vi "Configure Clock Recovery Method.vi"(0 "VISA resource name":refnum<visa-resource-name>, 1 "Clock":T1 {"Clock Edge (0: Rising)" items=["Rising", "Falling", "Both"]}, 2 "Track Frequency (2.5E+9 Hz)":dbl, 5 "Measurement Source (1: Channel 1)":i32(ring) items=["Channel 1", "Channel 2", "Channel 3", "Channel 4", "Function 1", "Function 2", "Function 3", "Function 4", "Memory 1", "Memory 2", "Memory 3", "Memory 4"], 7 "Clock Recovery Method (4: Constant Frequency)":i32(ring) items=["PCI Express", "Fibre Channel", "First Order PLL", "Second Order PLL", "Constant Frequency", "Explicit Clock", "Explicit First Order PLL", "Explicit Second Order PLL"], 9 "Data Rate and Bandwidth":T2 {"Data Bits (0: Both)" items=["Both", "Deemphasis", "Transition"]; "Data Rate Type (0: Fully Automatic)" items=["Fully Automatic", "Semi-Automatic", "Manual"]}, 11 "error in (no error)":errorcluster, 12 "Fibre Channel (0: FC1063)":i32(ring) items=["FC1063", "FC2125", "FC425"], 13 "Damping Factor (1 bits/s)":dbl format="%#.3g") -> (4 "VISA resource name out":refnum<visa-resource-name>, 15 "error out":errorcluster)   [LabVIEW 2009, in "Agilent 8000 Series.lvlib"]
doc: "Configures the clock recovery method parameters."
uses:
  Agilent 8000 Series.lvlib
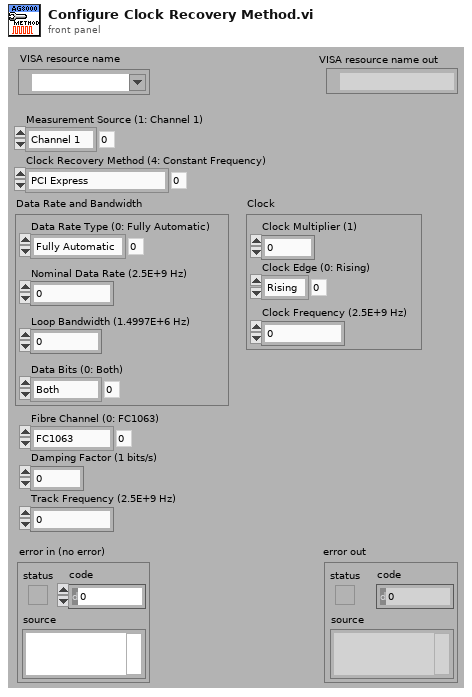
[diagram p1: front panel]
types:
  T1 = cluster{"Clock Edge (0: Rising)":i32, "Clock Multiplier (1)":i32, "Clock Frequency (2.5E+9 Hz)":dbl}
  T2 = cluster{"Nominal Data Rate (2.5E+9 Hz)":dbl, "Loop Bandwidth (1.4997E+6 Hz)":dbl, "Data Rate Type (0: Fully Automatic)":i32, "Data Bits (0: Both)":i32}
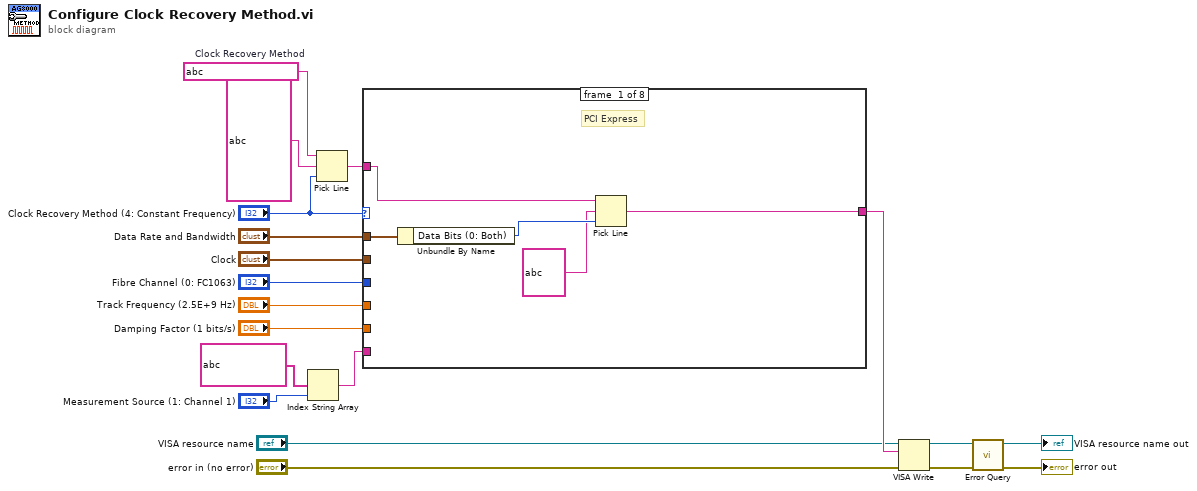
[diagram p0: block diagram]
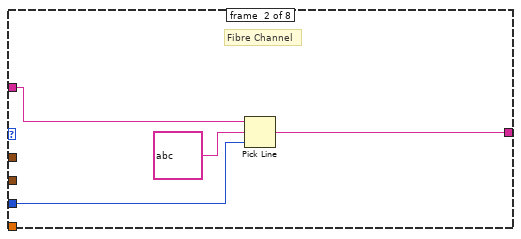
[diagram p2: hidden frame]
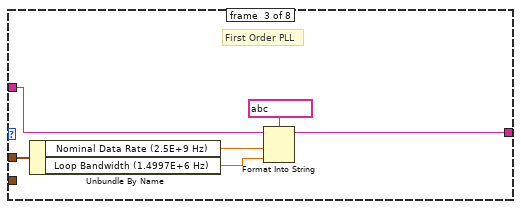
[diagram p3: hidden frame]
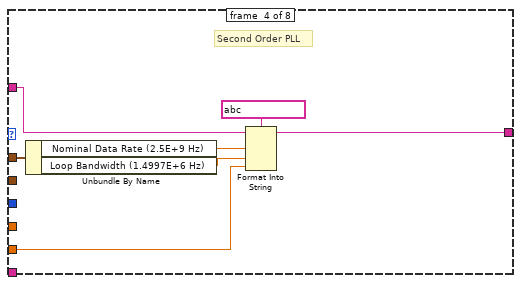
[diagram p4: hidden frame]
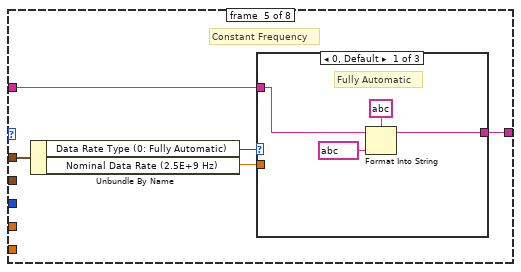
[diagram p5: hidden frame]
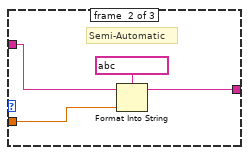
[diagram p6: hidden frame]
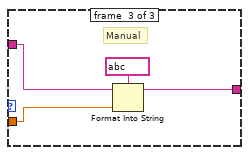
[diagram p7: hidden frame]
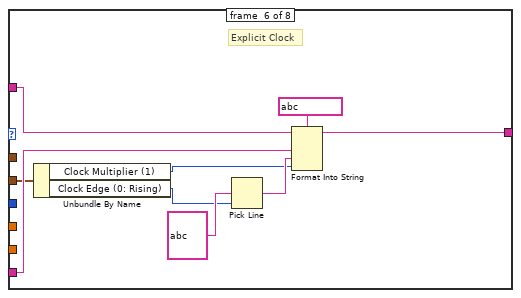
[diagram p8: hidden frame]
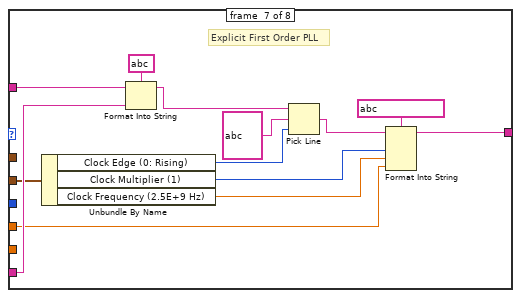
[diagram p9: hidden frame]
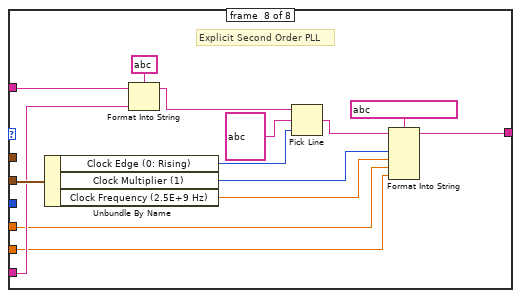
[diagram p10: hidden frame]
diagram:
  w19 = string ?  # Clock Recovery Method
  n1 = Index String Array(1:"Measurement Source (1: Channel 1)", 2:string[] ?) -> (0:w1:string)  [unwired: 1 in]
  n2 = Pick Line(string ("")=w19, multi-line string=string ?, line index="Clock Recovery Method (4: Constant Frequency)") -> (output string=w16:string)
  n3 = case shown="4" "Clock Recovery Method (4: Constant Frequency)" {
    tunnel: w16 -> [w23 w27 w33 w39 w44 w67 w78 w86]
    tunnel: "Data Rate and Bandwidth" -> [w24 _ w32 w40 w46 _ _ _]
    tunnel: [w20 w28 w34 w41 w43 w61 w72 w85] -> w10
    tunnel: "Clock" -> [_ _ _ _ _ w64 w75 w84]
    tunnel: "Fibre Channel (0: FC1063)" -> [_ w26 _ _ _ _ _ _]
    tunnel: "Track Frequency (2.5E+9 Hz)" -> [_ _ _ _ _ _ w68 w82]
    tunnel: "Damping Factor (1 bits/s)" -> [_ _ _ w35 _ _ _ w81]
    tunnel: w1 -> [_ _ _ _ _ w65 w79 w83]
    frame #0 {
      # "PCI Express"
      n4 = Unbundle By Name(w24) -> ("Data Bits (0: Both)"=w22:i32)
      n5 = Pick Line(string ("")=w23, multi-line string=string ? ("string (\"\")"), line index=w22) -> (output string=w20:string)
    }
    frame #1 {
      # "Fibre Channel"
      n6 = Pick Line(string ("")=w27, multi-line string=string ?, line index=w26) -> (output string=w28:string)
    }
    frame #2 {
      # "First Order PLL"
      n7 = Unbundle By Name(w32) -> ("Nominal Data Rate (2.5E+9 Hz)"=w30:dbl, "Loop Bandwidth (1.4997E+6 Hz)"=w29:dbl)
      n8 = Format Into String(format string=string ?, initial string=w33, w30, w29) -> (resulting string=w34:string)  [unwired: 1 in, 1 out]
    }
    frame #3 {
      # "Second Order PLL"
      n9 = Unbundle By Name(w40) -> ("Nominal Data Rate (2.5E+9 Hz)"=w37:dbl, "Loop Bandwidth (1.4997E+6 Hz)"=w36:dbl)
      n10 = Format Into String(format string=string ?, initial string=w39, w37, w36, w35) -> (resulting string=w41:string)  [unwired: 1 in, 1 out]
    }
    frame #4 {
      # "Constant Frequency"
      n11 = Unbundle By Name(w46) -> ("Data Rate Type (0: Fully Automatic)"=w45:i32, "Nominal Data Rate (2.5E+9 Hz)"=w42:dbl)
      n12 = case shown="0, Default" w45 {
        tunnel: w44 -> [w49 w53 w56]
        tunnel: [w50 w54 w55] -> w43
        tunnel: w42 -> [_ w51 w57]
        frame #0 {
          # "Fully Automatic"
          n13 = Format Into String(format string=string ?, initial string=w49, string ? ("input 1")) -> (resulting string=w50:string)  [unwired: 1 in, 1 out]
        }
        frame #1 {
          # "Semi-Automatic"
          n14 = Format Into String(format string=string ?, initial string=w53, w51) -> (resulting string=w54:string)  [unwired: 1 in, 1 out]
        }
        frame #2 {
          # "Manual"
          n15 = Format Into String(format string=string ?, initial string=w56, w57) -> (resulting string=w55:string)  [unwired: 1 in, 1 out]
        }
      }
    }
    frame #5 {
      # "Explicit Clock"
      n16 = Unbundle By Name(w64) -> ("Clock Multiplier (1)"=w60:i32, "Clock Edge (0: Rising)"=w59:i32)
      n17 = Pick Line(multi-line string=string ?, line index=w59) -> (output string=w63:string)  [unwired: 1 in]
      n18 = Format Into String(format string=string ?, initial string=w67, w65, w63, w60) -> (resulting string=w61:string)  [unwired: 1 in, 1 out]
    }
    frame #6 {
      # "Explicit First Order PLL"
      n19 = Unbundle By Name(w75) -> ("Clock Edge (0: Rising)"=w74:i32, "Clock Multiplier (1)"=w70:i32, "Clock Frequency (2.5E+9 Hz)"=w69:dbl)
      n20 = Format Into String(format string=string ?, initial string=w78, w79) -> (resulting string=w77:string)  [unwired: 1 in, 1 out]
      n21 = Pick Line(string ("")=w77, multi-line string=string ?, line index=w74) -> (output string=w73:string)
      n22 = Format Into String(format string=string ?, initial string=w73, w70, w69, w68) -> (resulting string=w72:string)  [unwired: 1 in, 1 out]
    }
    frame #7 {
      # "Explicit Second Order PLL"
      n23 = Unbundle By Name(w84) -> ("Clock Edge (0: Rising)"=w90:i32, "Clock Multiplier (1)"=w93:i32, "Clock Frequency (2.5E+9 Hz)"=w94:dbl)
      n24 = Format Into String(format string=string ?, initial string=w86, w83) -> (resulting string=w88:string)  [unwired: 1 in, 1 out]
      n25 = Pick Line(string ("")=w88, multi-line string=string ?, line index=w90) -> (output string=w91:string)
      n26 = Format Into String(format string=string ?, initial string=w91, w93, w94, w82, w81) -> (resulting string=w85:string)  [unwired: 1 in, 1 out]
    }
  }
  n27 = VISA Write(VISA resource name="VISA resource name", write buffer=w10, error in (no error)="error in (no error)") -> (VISA resource name out=w7:refnum<visa-resource-name>, error out=w6:errorcluster)  [unwired: 1 out]
  n28 = call "Error Query.vi"("error in (no error)"=w6, "VISA resource name"=w7) -> ("error out"=→"error out":errorcluster, "VISA resource name out"=→"VISA resource name out":refnum<visa-resource-name>)  [unwired: 6 in, 2 out]
